vi "JournalDosimétrie.vi"() -> ()   [LabVIEW 2014]
doc: "Use this template to build a producer/consumer design pattern with events to produce queue items. Use this design pattern instead of the User Interface Event Handler pattern for user interfaces when you want to execute code asynchronously in response to an event without slowing the user interface responsiveness."
uses:
  Controls/Command.ctl
panel:
  in  "Resume":bool
  in  "Pause":bool
  out "Paused":bool
  out "Journal Path error out":errorcluster
  in  "Journal Path":path
  in  "Journal Name":path=path "Journal_AT1123.dat"
  out "Started":bool
  out "VISA error out":errorcluster
  in  "VISA error in (no error)":errorcluster
  in  "baud rate":u32=9600
  in  "VISA resource name":refnum<visa-resource-name>="COM1"
  out "Débit de Dose":dbl(graph)
  out "Dose":dbl(graph)
  in  "Start Journaling":bool
  in  "stop":bool
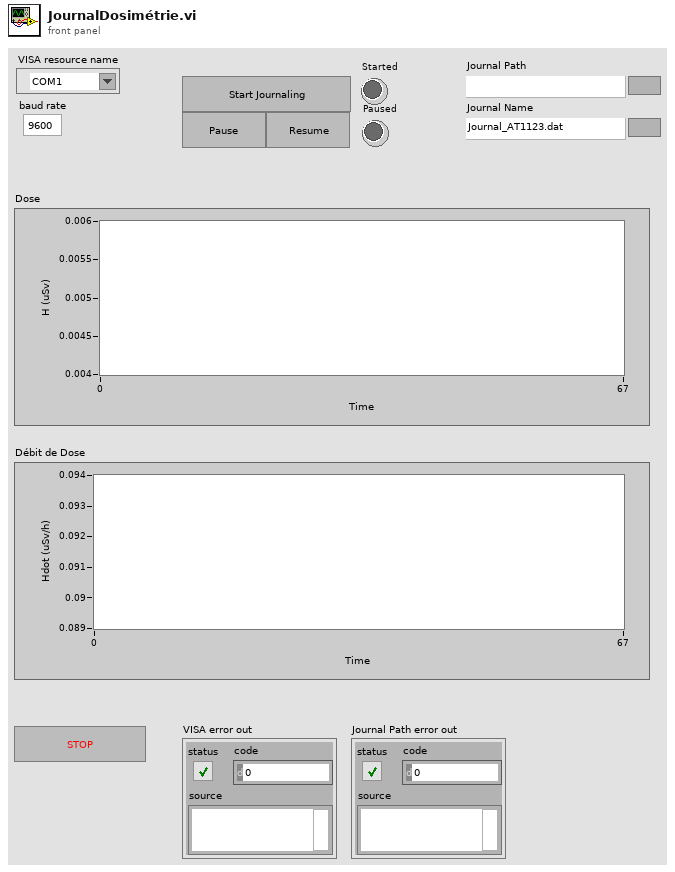
[diagram p1: front panel]
types:
  T1 = enum16{"open", "replace", "create", "open or create", "replace or create", "replace or create with confirmation"}
  T2 = typedef "Command.ctl" = enum16{"Get Data", "Do nothing", "Stop Programme", "Resume", "Pause", "Get Max Hdot", "Get Max H", "Start Journaling"}
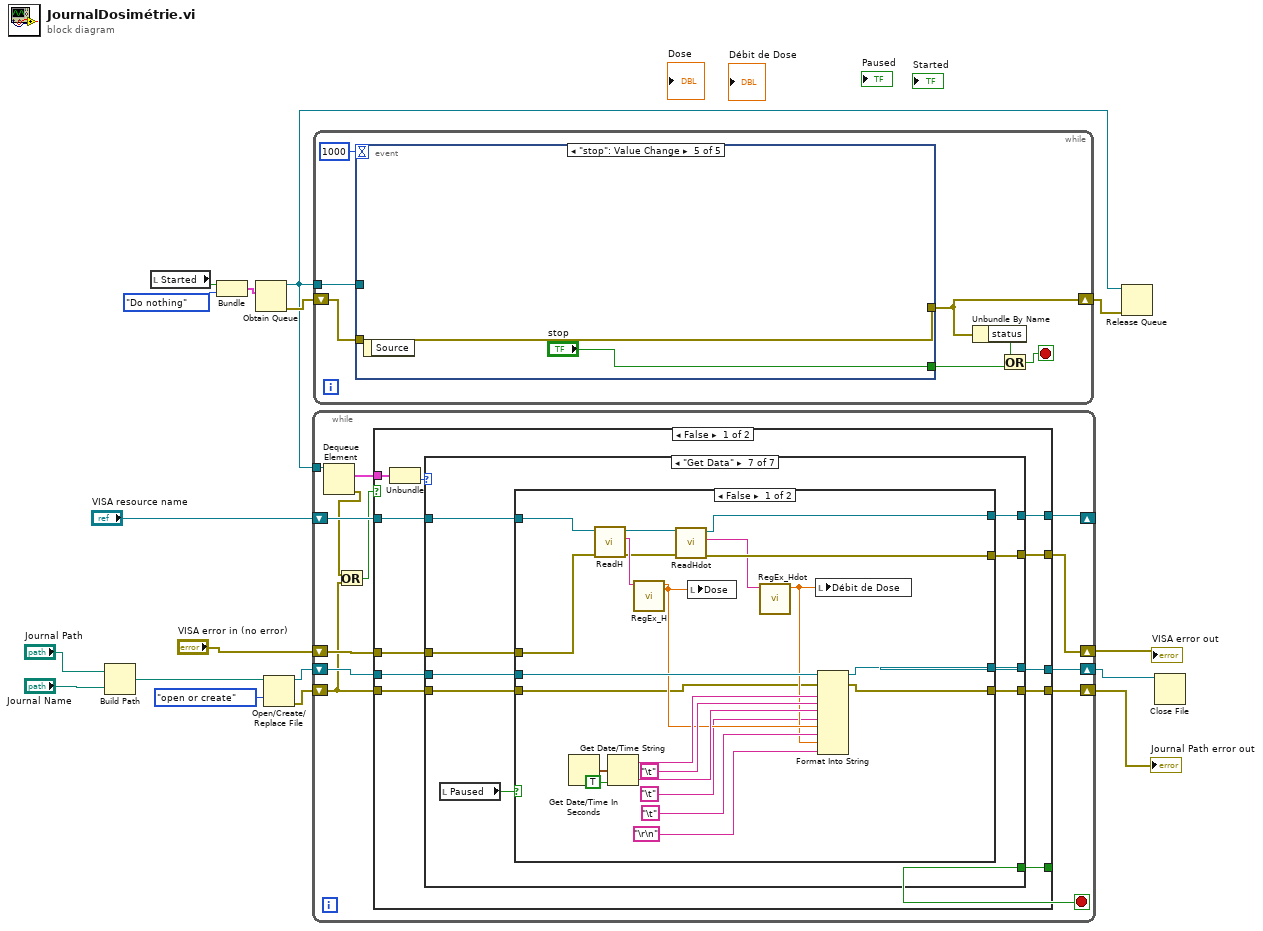
[diagram p0: block diagram]
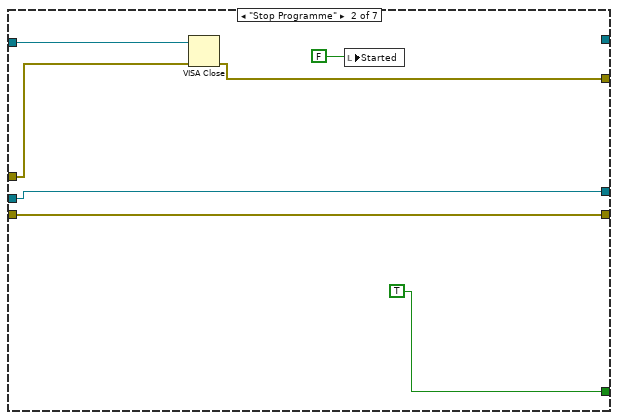
[diagram p3: hidden frame]
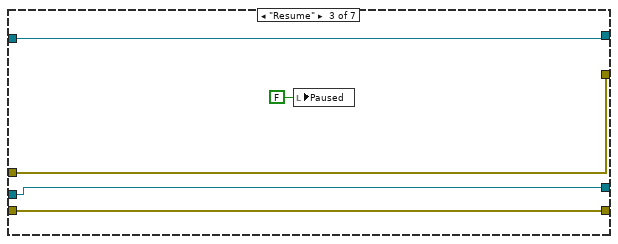
[diagram p4: hidden frame]
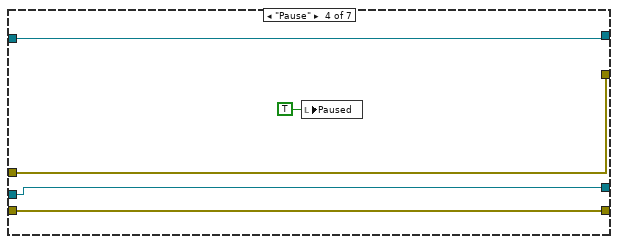
[diagram p5: hidden frame]
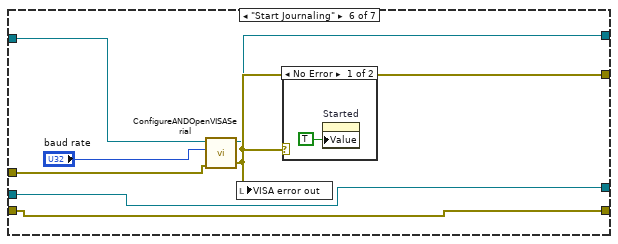
[diagram p7: hidden frame]
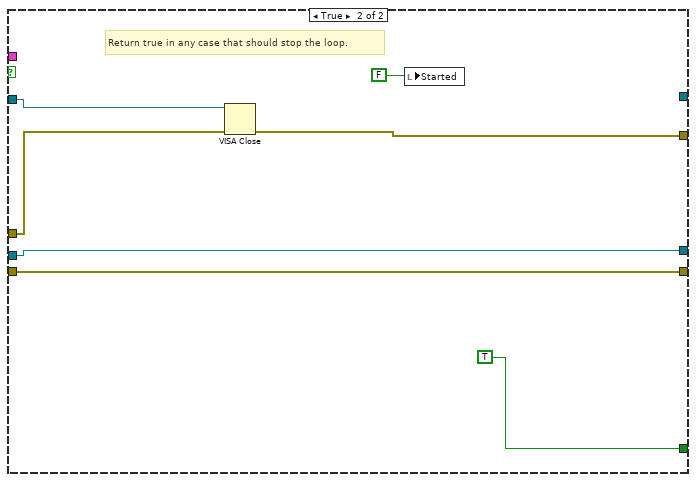
[diagram p10: hidden frame]
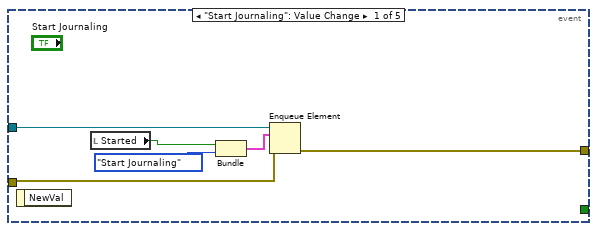
[diagram p11: hidden frame]
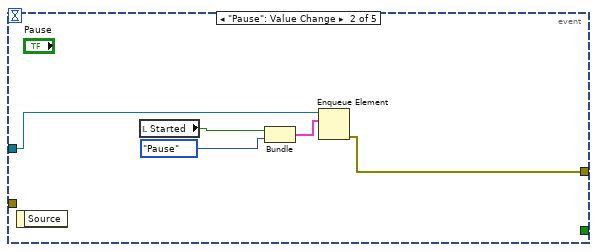
[diagram p12: hidden frame]
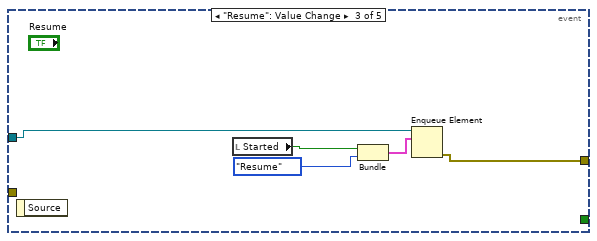
[diagram p13: hidden frame]
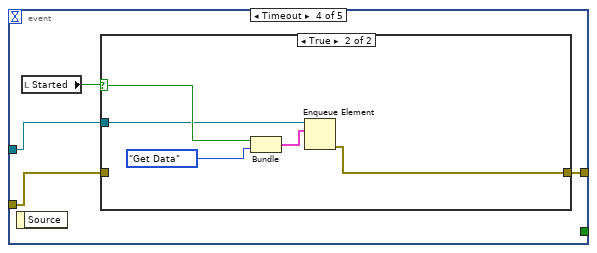
[diagram p14: hidden frame]
diagram:
  n1 = Build Path(base path="Journal Path", name or relative path="Journal Name") -> (appended path=w7:path)
  n2 = local read "Started"() -> (w9:bool)
  n3 = Bundle("Started"=w9, "Command"=Command."Do nothing") -> (w10:cluster{"Started":bool, "Command":T2})  [unwired: 1 in]
  n4 = Obtain Queue(element data type=w10) -> (queue out=w15:refnum<queue>, error out=w17:errorcluster)  [unwired: 4 in, 1 out]
  n5 = Open/Create/Replace File(file path (use dialog)=w7, operation (0:open)=T1."open or create") -> (refnum out=w5:refnum<file>, error out=w4:errorcluster)  [unwired: 4 in, 1 out]
  n6 = while {
    tunnel: w15 -> [w30]
    shift-right: [w26] -> w13
    shift-left: "VISA error in (no error)" -> [w27]
    shift-right: [w24] -> _
    shift-left: "VISA resource name" -> [w25]
    shift-right: [w22] -> w2
    shift-left: w5 -> [w23]
    shift-right: [w21] -> w3
    shift-left: w4 -> [w20]
    stop <- w28 stop-if-true
    n7 = Dequeue Element(queue=w30) -> (element=w29:cluster{"Started":bool, "Command":T2}, error out=w19:errorcluster)  [unwired: 2 in, 2 out]
    n8 = Or(x=w19, y=w20) -> (x .or. y?=w18:bool)
    n9 = case shown="False" w18 {
      tunnel: w29 -> [w39 _]
      tunnel: [w35 TRUE] -> w28
      tunnel: w27 -> [w41 w114]
      tunnel: [w40 w113] -> w26
      tunnel: w25 -> [w37 w115]
      tunnel: [w36 _] -> w24
      tunnel: w23 -> [w34 w111]
      tunnel: [w33 w111] -> w22
      tunnel: w20 -> [w32 w110]
      tunnel: [w31 w110] -> w21
      frame False {
        n10 = Unbundle(w39) -> ("Command"=w38:T2)  [unwired: 1 out]
        n11 = case shown="\"Get Data\"" w38 {
          tunnel: w41 -> [w44 w51 w56 w61 w65 w72 w82]
          tunnel: [w44 w50 w56 w61 w65 w71 w80] -> w40
          tunnel: [w45 _ w57 w62 w66 w70 w81] -> w36
          tunnel: w37 -> [w45 w52 w57 w62 w66 w69 w83]
          tunnel: [_ TRUE _ _ _ _ _] -> w35
          tunnel: w34 -> [w42 w47 w55 w60 w64 w68 w79]
          tunnel: [w42 w47 w55 w60 w64 w68 w78] -> w33
          tunnel: w32 -> [w43 w46 w54 w59 w63 w67 w77]
          tunnel: [w43 w46 w54 w59 w63 w67 w76] -> w31
          frame "Do nothing", Default {
          }
          frame "Stop Programme" {
            n12 = VISA Close(VISA resource name=w52, error in (no error)=w51) -> (error out=w50:errorcluster)
            n13 = local write "Started"(FALSE) -> ()
          }
          frame "Resume" {
            n14 = local write "Paused"(FALSE ("Paused")) -> ()
          }
          frame "Pause" {
            n15 = local write "Paused"(TRUE ("Paused")) -> ()
          }
          frame "Get Max Hdot" {
          }
          frame "Start Journaling" {
            n16 = call "ConfigureANDOpenVISASerial.vi"("error in (no error)"=w72, "baud rate (9600)"="baud rate", "VISA resource name"=w69) -> ("error out"=w71:errorcluster, "VISA resource name out"=w70:refnum<visa-resource-name>)  [unwired: 7 in]
            n17 = local write "VISA error out"(w71) -> ()
            n18 = case shown="No Error" w71 {
              frame No Error {
                n19 = property on="Started" class="Bool (strict)"("Value"=TRUE ("Started")) -> ()  [unwired: 2 in, 2 out]
              }
              frame Error {
              }
            }
          }
          frame "Get Data" {
            n20 = local read "Paused"() -> (w75:bool)
            n21 = case shown="False" w75 {
              tunnel: w83 -> [w105 w109]
              tunnel: w82 -> [w104 w108]
              tunnel: [w100 w109] -> w81
              tunnel: [w99 w108] -> w80
              tunnel: w79 -> [w96 w107]
              tunnel: [w88 w107] -> w78
              tunnel: w77 -> [w86 w106]
              tunnel: [w85 w106] -> w76
              frame False {
                n22 = Get Date/Time In Seconds() -> (seconds since 1Jan1904=w97:timestamp)
                n23 = call "ReadH.vi"("error in (no error)"=w104, "VISA Refnum in"=w105) -> ("error out"=w101:errorcluster, "read buffer"=w103:string, "VISA Refnum out"=w102:refnum<visa-resource-name>)  [unwired: 7 in]
                n24 = Get Date/Time String(seconds (now)=w97, want seconds? (F)=TRUE) -> (date string=w95:string, time string=w93:string)  [unwired: 1 in]
                n25 = call "RegEx_H.vi"("H String"=w103) -> ("H dbl (uSv)"=w92:dbl)  [unwired: 9 in, 1 out]
                n26 = call "ReadHdot.vi"("error in (no error)"=w101, "VISA Refnum in"=w102) -> ("error out"=w99:errorcluster, "read buffer"=w98:string, "VISA Refnum out"=w100:refnum<visa-resource-name>)  [unwired: 7 in]
                n27 = local write "Dose"(w92) -> ()
                n28 = call "RegEx_Hdot.vi"("Hdot String"=w98) -> ("Hdot dbl (uSv/s)"=w90:dbl)  [unwired: 9 in, 1 out]
                n29 = local write "Débit de Dose"(w90) -> ()
                n30 = Format Into String(initial string=w96, error in=w86, w95, "\t", w93, "\t", w92, "\t", w90, "\r\n") -> (resulting string=w88:refnum<file>, error out=w85:errorcluster)  [unwired: 1 in]
              }
              frame True {
              }
            }
          }
        }
      }
      frame True {
        # "Return true in any case that should stop the loop."
        n31 = VISA Close(VISA resource name=w115, error in (no error)=w114) -> (error out=w113:errorcluster)
        n32 = local write "Started"(FALSE) -> ()
      }
    }
  }
  "VISA error out" <- w13
  "Journal Path error out" <- w3
  n33 = while {
    shift-right: [w119] -> w16
    shift-left: w17 -> [w122]
    tunnel: w15 -> [w123]
    stop <- w120 stop-if-true
    n34 = event shown="[4] \"stop\": Value Change" {
      selector: _ -> [_ _ _ _ _]
      dyn-events: _ -> [_ _ _ _ _]
      timeout: 1000 -> [_ _ _ _ _]
      tunnel: w123 -> [w129 w132 w136 w140 _]
      tunnel: w122 -> [w128 _ _ w141 w150]
      tunnel: [w127 w130 w135 w142 w150] -> w119
      tunnel: [_ _ _ _ "stop"] -> w121
      event "Start Journaling": Value Change {
        n35 = event-data() -> ()  [unwired: 1 in, 1 out]
        n36 = local read "Started"() -> (w126:bool)
        n37 = Bundle("Started"=w126, "Command"=Command."Start Journaling") -> (w124:cluster{"Started":bool, "Command":T2})  [unwired: 1 in]
        n38 = Enqueue Element(queue=w129, element=w124, error in (no error)=w128) -> (error out=w127:errorcluster)  [unwired: 1 in, 2 out]
      }
      event "Pause": Value Change {
        n39 = event-data() -> ()  [unwired: 1 in, 1 out]
        n40 = local read "Started"() -> (w131:bool)
        n41 = Bundle("Started"=w131, "Command"=Command."Pause") -> (w133:cluster{"Started":bool, "Command":T2})  [unwired: 1 in]
        n42 = Enqueue Element(queue=w132, element=w133) -> (error out=w130:errorcluster)  [unwired: 2 in, 2 out]
      }
      event "Resume": Value Change {
        n43 = event-data() -> ()  [unwired: 1 in, 1 out]
        n44 = local read "Started"() -> (w137:bool)
        n45 = Bundle("Started"=w137, "Command"=Command."Resume") -> (w138:cluster{"Started":bool, "Command":T2})  [unwired: 1 in]
        n46 = Enqueue Element(queue=w136, element=w138) -> (error out=w135:errorcluster)  [unwired: 2 in, 2 out]
      }
      event Timeout {
        n47 = event-data() -> ()  [unwired: 1 in, 1 out]
        n48 = local read "Started"() -> (w143:bool)
        n49 = case shown="True" w143 {
          selector: w143 -> [_ w146]
          tunnel: [w144 w147] -> w142
          tunnel: w141 -> [w144 _]
          tunnel: w140 -> [_ w145]
          frame False {
          }
          frame True {
            n50 = Bundle(w146, "Command"=Command."Get Data") -> (w148:cluster{bool, "Command":T2})  [unwired: 1 in]
            n51 = Enqueue Element(queue=w145, element=w148) -> (error out=w147:errorcluster)  [unwired: 2 in, 2 out]
          }
        }
      }
      event "stop": Value Change {
        n52 = event-data() -> ()  [unwired: 1 in, 1 out]
      }
    }
    n53 = Unbundle By Name(w119) -> ("status"=w118:bool)
    n54 = Or(x=w118, y=w121) -> (x .or. y?=w120:bool)
  }
  n55 = Release Queue(queue=w15, error in (no error)=w16) -> ()  [unwired: 1 in, 3 out]
  n56 = Close File(refnum=w2) -> ()  [unwired: 1 in, 2 out]
